vi "FTW-Endpoint-Multipart-Ask.vi"(0 "FTW Endpoint":refnum<class "FTW-Endpoint.lvclass">, 5 "Multipart Message":string[](array[string]), 7 "Read Timeout":i32=100 format="%dmsec", 9 "Write Timeout":i32 format="%dmsec", 11 "error in":errorcluster) -> (4 "FTW Endpoint out":refnum<class "FTW-Endpoint.lvclass">, 6 "Reply":string[](array[string]), 8 "Read Timed out?":bool, 10 "Write Timed out?":bool, 15 "error out":errorcluster)   [LabVIEW 2012, in "FTW-Actor.lvlib" / "FTW-Endpoint.lvclass"]
uses:
  FTW-Endpoint.lvclass
  Ether/FTW-Ether.lvclass
panel:
  # "Inputs"
  # "Outputs"
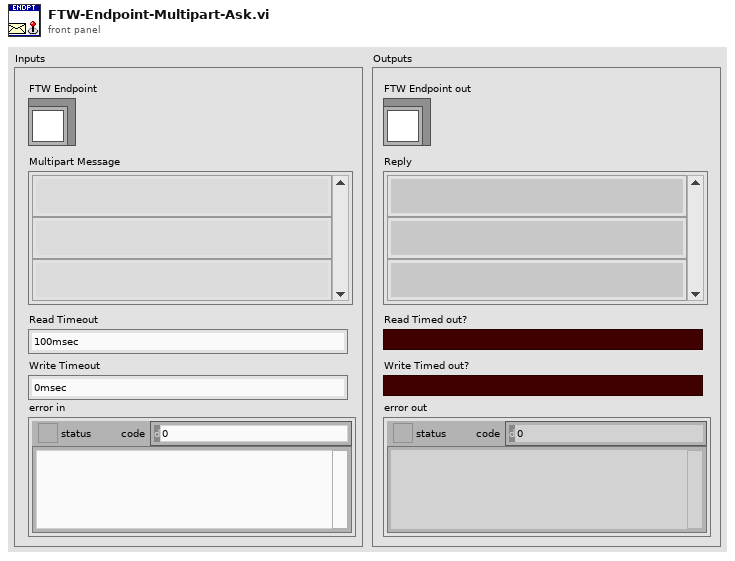
[diagram p1: front panel]
types:
  T1 = typedef "FTW-Actor.lvlib/FTW-Actor-Address.ctl" = string
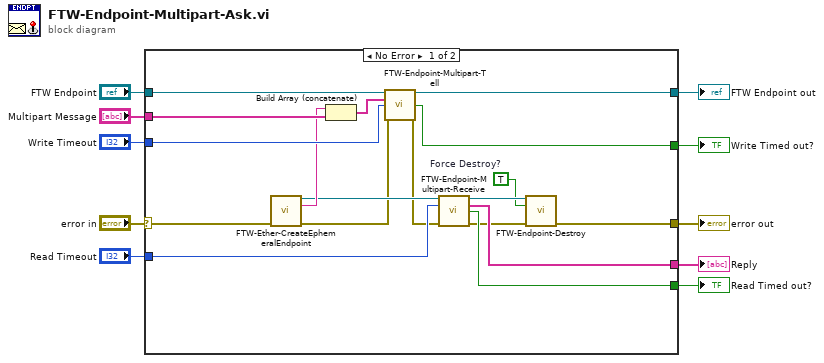
[diagram p0: block diagram]
diagram:
  n1 = case shown="No Error" "error in" {
    selector: "error in" -> [w22 w30]
    tunnel: [w12 w30] -> w10
    tunnel: [w25 w29] -> w8
    tunnel: "FTW Endpoint" -> [w26 w29]
    tunnel: "Multipart Message" -> [w28 _]
    tunnel: "Read Timeout" -> [w19 _]
    tunnel: [w16 _] -> w4
    tunnel: [w17 _] -> w3
    tunnel: [w24 _] -> w2
    tunnel: "Write Timeout" -> [w23 _]
    frame No Error {
      w14 = TRUE  # Force Destroy?
      n2 = call "FTW-Ether-CreateEphemeralEndpoint.vi"("error in"=w22) -> ("Ephemeral Endpoint"=w20:refnum<class "FTW-Endpoint.lvclass">, "Actual Ephemeral Address"=w21:T1, "error out"=w11:errorcluster)  [unwired: 12 in]
      n3 = Build Array (concatenate)(w21, w28) -> (w27:T1[])
      n4 = call-dynamic "FTW-Endpoint-Multipart-Tell.vi"("FTW Endpoint"=w26, "Multipart Message"=w27, "Timeout"=w23, "error in"=w11) -> ("FTW Endpoint out"=w25:refnum<class "FTW-Endpoint.lvclass">, "Timed out?"=w24:bool, "error out"=w18:errorcluster)  [unwired: 9 in]
      n5 = call-dynamic "FTW-Endpoint-Multipart-Receive.vi"("FTW Endpoint"=w20, "Timeout"=w19, "error in"=w18) -> ("FTW Endpoint out"=w15:refnum<class "FTW-Endpoint.lvclass">, "Message Received"=w17:string[], "Timed out?"=w16:bool, "error out"=w13:errorcluster)  [unwired: 9 in]
      n6 = call-dynamic "FTW-Endpoint-Destroy.vi"("FTW Endpoint"=w15, "Force Destroy"=w14, "error in"=w13) -> ("error out"=w12:errorcluster)  [unwired: 12 in]
    }
    frame Error {
    }
  }
  "error out" <- w10
  "FTW Endpoint out" <- w8
  "Read Timed out?" <- w4
  "Reply" <- w3
  "Write Timed out?" <- w2
